vi "SNF_Analog.vi"() -> ()   [LabVIEW 2017]
uses:
  Users/Darcy/Documents/LabVIEW Data/MathScriptVIs/MCStatic_38597428832_1f828b6118eee4aae6c26f87bca7dc42.vi
  <instcachedir>/0/MCStatic_38597428832_1f828b6118eee4aae6c26f87bca7dc42_D4E3D0E3241540FEBE7742005F22DD6C.lvgen/MCStatic_38597428832_1f828b6118eee4aae6c26f87bca7dc42_D4E3D0E3241540FEBE7742005F22DD6C_001.vi
  <vilib>/imath/engines/lvmath2/RunTimeEngine/IndexRead/NIMS V(S).vi
  <instcachedir>/0/NIMS V(S)_0488751826AF41519A22953C041130DC.lvgen/NIMS V(S)_0488751826AF41519A22953C041130DC_000.vi
  <vilib>/imathl/engines/lvmath/Functions/Error Handling/Create Error.vi
  <vilib>/imath/engines/lvmath2/RunTimeEngine/NodeEndStatement/NIMS_NodeEndStatement_Output.vi
  <instcachedir>/0/NIMS_NodeEndStatement_Output_53EC0D466D134D7ABD903AC30B43404B.lvgen/NIMS_NodeEndStatement_Output_53EC0D466D134D7ABD903AC30B43404B_001.vi
  <instcachedir>/0/NIMS_NodeEndStatement_Output_53EC0D466D134D7ABD903AC30B43404B.lvgen/NIMS_NodeEndStatement_Output_53EC0D466D134D7ABD903AC30B43404B_005.vi
  <vilib>/imath/engines/lvmath2/RunTimeEngine/ErrorHandling/NIMS_Finalize Error.vi
  <vilib>/Utility/file.llb/Read Delimited Spreadsheet (DBL).vi
  Users/Darcy/Documents/LabVIEW Data/reactor_power.m
  Users/Darcy/Documents/LabVIEW Data/long_term_power.m
  Users/Darcy/Documents/LabVIEW Data/power_function.m
  Users/Darcy/Documents/LabVIEW Data/short_term_power.m
panel:
  out "Coolant Temp\n Avg.":dbl
  in  "dt (milliseconds)":i64=50
  in  "CRsteady":dbl=50.0 format="%#_13g"
  in  "CRamp":dbl=200.0
  in  "power":dbl=50.0 format="%#_13g"
  in  "P_max: 100":dbl=200.0
  in  "P_min: 1":dbl=1.0
  out "ST Avg.":dbl
  out "Coolant Temp":dbl(slide) scale=20.0..100.0
  out "Fuel Temp":dbl(slide) scale=100.0..175.0
  out "BT Avg.":dbl
  out "CX Avg.":dbl
  in  "Input Length":dbl
  out "Iterations":dbl
  in  "?":bool
  in  "?":bool
  out "Array":dbl[](array[numeric])
  in  "INPUT/MANUAL":bool
  in  "Load Power Profile":bool
  in  "Dyn. Control Rod Profile File":path
  in  "?":bool
  in  "Equilibrium T_Coolant\nFHR: 100":dbl=100.0
  in  "Equilibrium T_Fuel\nFHR: 100":dbl=100.0
  in  "Coolant Feedback Coef\nFHR: -2.1":dbl=-2.1
  in  "Fuel Feedback Coef\nFHR: -6.7":dbl=-6.7
  in  "CRW Coef":dbl=0.005
  in  "CRW Constant":dbl=0.997
  in  "beta\nFHR: 0.0065":dbl=0.0065
  in  "Lambda\nFHR: 5.02e-4":dbl=0.000502
  in  "lambda\nFHR: 0.0785":dbl=0.0785
  out "Net Reactivity":dbl
  out "Rod Reactivity":dbl
  out "Rod 1 In":dbl(slide)
  out "Rod 1 Out":dbl(slide) scale=0.0..1.0
  out "?":dbl(slide) scale=1.0..10000.0
  out "Net Amount Rod Out":dbl
  out "Power [W]":dbl
  in  "SCRAM":bool
  out "Power":dbl(graph)
  out "Resolution 1":dbl=0.05
  out "Control Rod 1 Out":dbl=0.6
  in  "STOP TOGGLE":bool
  # "Neutronics"
  # "Control Rod Worth (CRW)"
  # "Outside Core"
  # "Inside Core"
  # "Temperature Feedback"
  # "Fine"
  # "Input"
  # "Manual"
  # "Coarse"
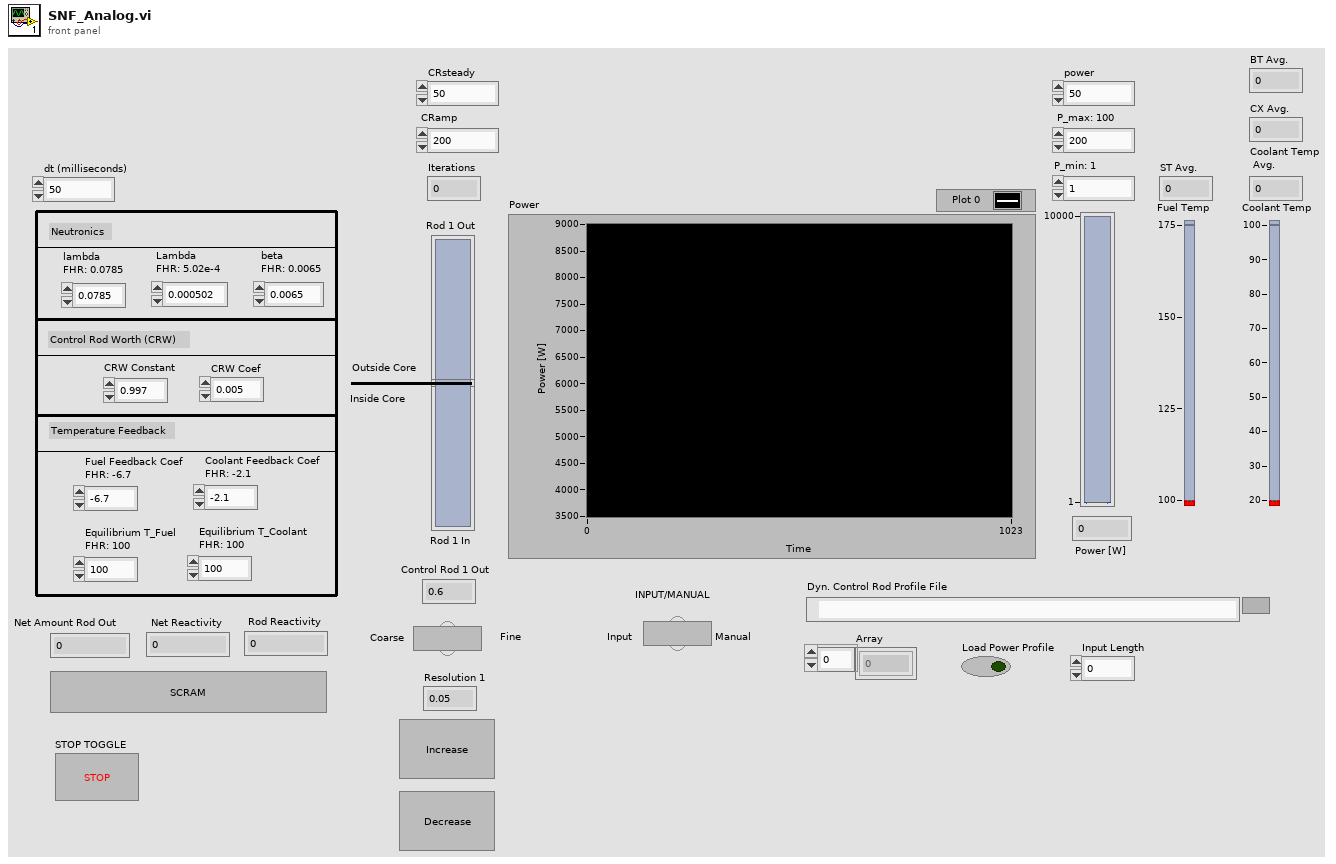
[diagram p1: front panel]
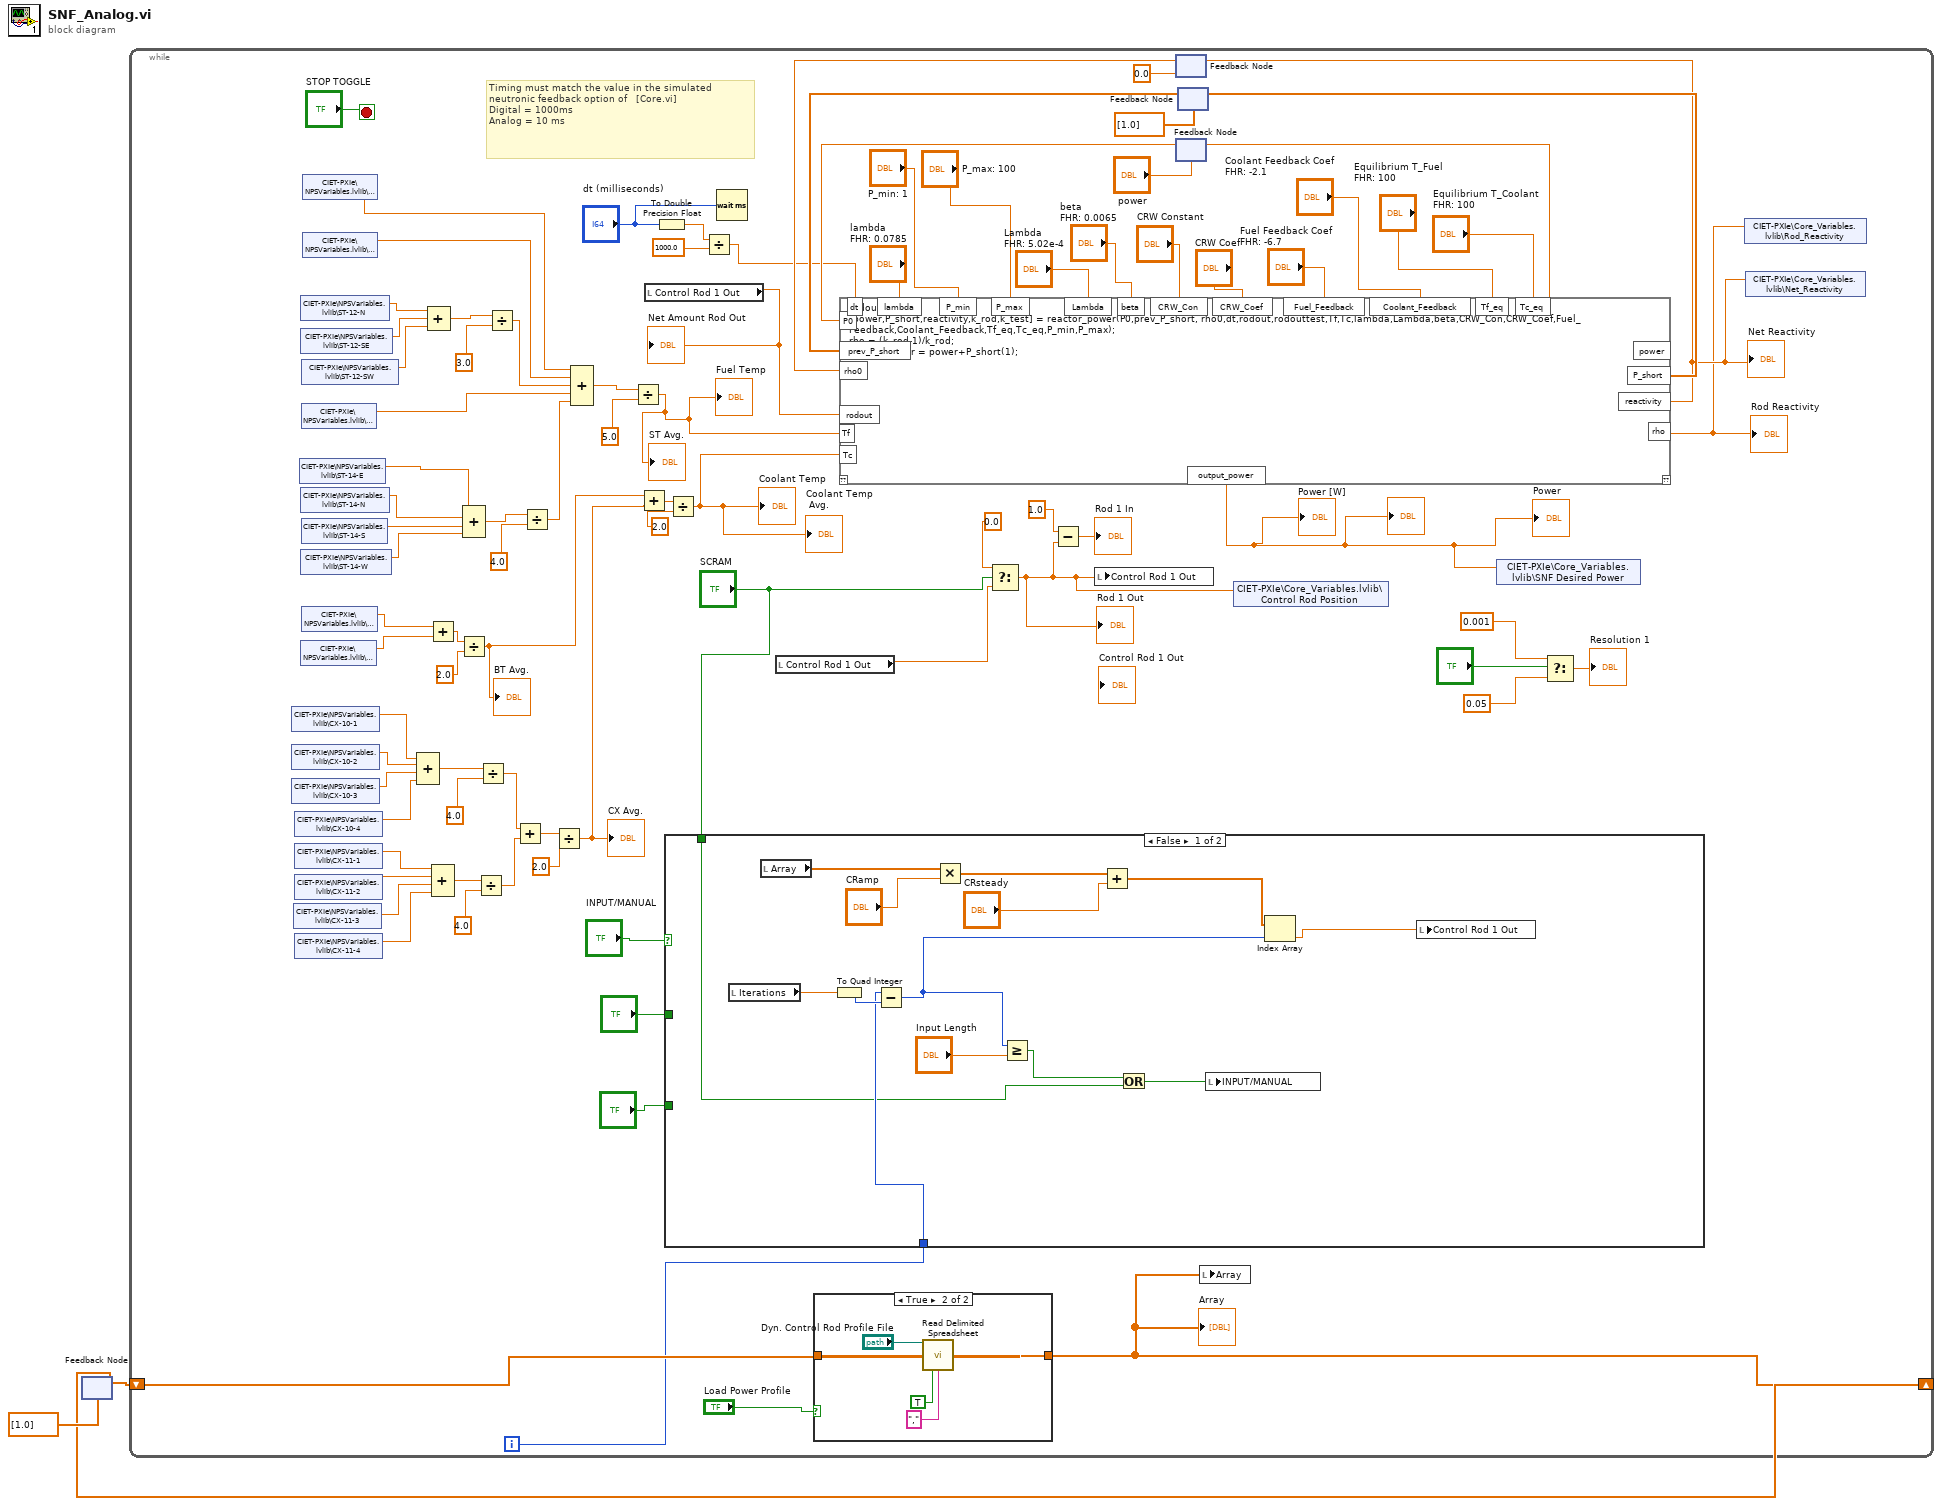
[diagram p0: block diagram]
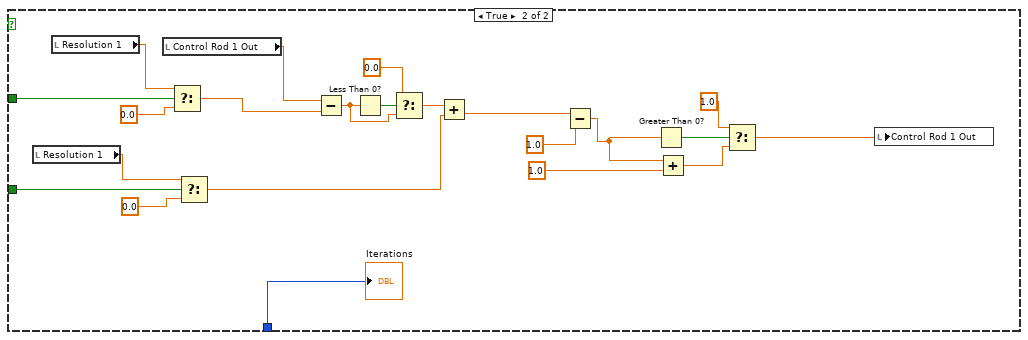
[diagram p2: hidden frame]
diagram:
  n1 = feedback #1(dbl[] [1.0] ("P_short")) -> (w3:dbl[])
  n2 = while {
    shift-right: [w64] -> w1
    shift-left: w3 -> [w65]
    i -> [w59]
    stop <- "STOP TOGGLE" stop-if-true
    # "Timing must match the value in the simulated neutronic feedback option of   [Core.vi] \nDigital = 1000ms \nAnalog = 10 ms"
    n3 = shared-variable "CIET-PXIe\\NPSVariables.lvlib\\CX-10-1"() -> (w24:sgl)  [unwired: 1 in, 1 out]
    n4 = shared-variable "CIET-PXIe\\NPSVariables.lvlib\\CX-10-2"() -> (w23:sgl)  [unwired: 1 in, 1 out]
    n5 = shared-variable "CIET-PXIe\\NPSVariables.lvlib\\CX-10-3"() -> (w22:sgl)  [unwired: 1 in, 1 out]
    n6 = shared-variable "CIET-PXIe\\NPSVariables.lvlib\\CX-11-3"() -> (w18:sgl)  [unwired: 1 in, 1 out]
    n7 = shared-variable "CIET-PXIe\\NPSVariables.lvlib\\CX-10-4"() -> (w21:sgl)  [unwired: 1 in, 1 out]
    n8 = shared-variable "CIET-PXIe\\NPSVariables.lvlib\\CX-11-1"() -> (w20:sgl)  [unwired: 1 in, 1 out]
    n9 = shared-variable "CIET-PXIe\\NPSVariables.lvlib\\CX-11-2"() -> (w19:sgl)  [unwired: 1 in, 1 out]
    n10 = shared-variable "CIET-PXIe\\NPSVariables.lvlib\\CX-11-4"() -> (w17:sgl)  [unwired: 1 in, 1 out]
    n11 = shared-variable "CIET-PXIe\\NPSVariables.lvlib\\ST-14-E"() -> (w39:sgl)  [unwired: 1 in, 1 out]
    n12 = shared-variable "CIET-PXIe\\NPSVariables.lvlib\\ST-12-N"() -> (w46:sgl)  [unwired: 1 in, 1 out]
    n13 = shared-variable "CIET-PXIe\\NPSVariables.lvlib\\ST-12-SE"() -> (w45:sgl)  [unwired: 1 in, 1 out]
    n14 = shared-variable "CIET-PXIe\\NPSVariables.lvlib\\ST-14-N"() -> (w38:sgl)  [unwired: 1 in, 1 out]
    n15 = shared-variable "CIET-PXIe\\NPSVariables.lvlib\\ST-14-W"() -> (w36:sgl)  [unwired: 1 in, 1 out]
    n16 = shared-variable "CIET-PXIe\\NPSVariables.lvlib\\BT-12"() -> (w53:sgl)  [unwired: 1 in, 1 out]
    n17 = shared-variable "CIET-PXIe\\NPSVariables.lvlib\\ST-12-SW"() -> (w44:sgl)  [unwired: 1 in, 1 out]
    n18 = shared-variable "CIET-PXIe\\NPSVariables.lvlib\\ST-13"() -> (w42:sgl)  [unwired: 1 in, 1 out]
    n19 = shared-variable "CIET-PXIe\\NPSVariables.lvlib\\ST-14-S"() -> (w37:sgl)  [unwired: 1 in, 1 out]
    n20 = shared-variable "CIET-PXIe\\NPSVariables.lvlib\\BT-11"() -> (w54:sgl)  [unwired: 1 in, 1 out]
    n21 = shared-variable "CIET-PXIe\\NPSVariables.lvlib\\ST-10"() -> (w52:sgl)  [unwired: 1 in, 1 out]
    n22 = shared-variable "CIET-PXIe\\NPSVariables.lvlib\\ST-11"() -> (w51:sgl)  [unwired: 1 in, 1 out]
    n23 = Compound Arithmetic op=ADD(w24, w23, w22, w21) -> (w30:sgl)
    n24 = Compound Arithmetic op=ADD(w46, w45, w44) -> (w48:sgl)
    n25 = Add(x=w54, y=w53) -> (x+y=w56:sgl)
    n26 = Compound Arithmetic op=ADD(w20, w19, w18, w17) -> (w28:sgl)
    n27 = Divide(x=w56, y=2.0) -> (x/y=w33:dbl)
    "BT Avg." <- w33
    n28 = Compound Arithmetic op=ADD(w39, w38, w37, w36) -> (w41:sgl)
    n29 = Divide(x=w28, y=4.0) -> (x/y=w25:dbl)
    n30 = Divide(x=w30, y=4.0) -> (x/y=w26:dbl)
    n31 = Divide(x=w48, y=3.0) -> (x/y=w43:dbl)
    n32 = Add(x=w26, y=w25) -> (x+y=w58:dbl)
    n33 = Divide(x=w41, y=4.0) -> (x/y=w35:dbl)
    n34 = Divide(x=w58, y=2.0) -> (x/y=w32:dbl)
    "CX Avg." <- w32
    n35 = Compound Arithmetic op=ADD(w52, w51, w43, w42, w35) -> (w50:dbl)
    n36 = Divide(x=w50, y=5.0) -> (x/y=w16:dbl)
    "Fuel Temp" <- w16
    "ST Avg." <- w16
    n37 = Add(x=w33, y=w32) -> (x+y=w31:dbl)
    n38 = local read "Control Rod 1 Out"() -> (w67:dbl)
    "Net Amount Rod Out" <- w67
    n39 = To Double Precision Float(number="dt (milliseconds)") -> (double precision float=w7:dbl)
    n40 = case shown="False" "INPUT/MANUAL" {
      tunnel: "?" -> [_ w110]
      tunnel: "?" -> [_ w109]
      tunnel: w59 -> [w102 w108]
      tunnel: "SCRAM" -> [w100 _]
      frame False {
        n41 = local read "Iterations"() -> (w104:dbl)
        n42 = local read "Array"() -> (w97:dbl[])
        n43 = To Quad Integer(1:w104) -> (0:w103:i64)
        n44 = Subtract(x=w102, y=w103) -> (x-y=w105:i64)
        n45 = Multiply(x=w97, y="CRamp") -> (x*y=w95:dbl[])
        n46 = Greater Or Equal?(x=w105, y="Input Length") -> (x >= y?=w101:bool)
        n47 = Add(x=w95, y="CRsteady") -> (x+y=w93:dbl[])
        n48 = Or(x=w101, y=w100) -> (x .or. y?=w99:bool)
        n49 = local write "INPUT/MANUAL"(w99) -> ()
        n50 = Index Array(array=w93, index=w105) -> (element=w98:dbl)
        n51 = local write "Control Rod 1 Out"(w98) -> ()
      }
      frame True {
        n52 = local read "Resolution 1"() -> (w126:dbl)
        n53 = local read "Resolution 1"() -> (w128:dbl)
        n54 = local read "Control Rod 1 Out"() -> (w124:dbl)
        n55 = Select(t=w128, s=w110, f=0.0) -> (s? t:f=w123:dbl)
        n56 = Select(t=w126, s=w109, f=0.0) -> (s? t:f=w111:dbl)
        n57 = Subtract(x=w124, y=w123) -> (x-y=w121:dbl)
        n58 = Less Than 0?(x=w121) -> (x < 0?=w122:bool)
        n59 = Select(t=0.0, s=w122, f=w121) -> (s? t:f=w119:dbl)
        n60 = Add(x=w119, y=w111) -> (x+y=w118:dbl)
        n61 = Subtract(x=w118, y=1.0) -> (x-y=w114:dbl)
        n62 = Greater Than 0?(x=w114) -> (x > 0?=w116:bool)
        n63 = Add(x=w114, y=1.0) -> (x+y=w113:dbl)
        n64 = Select(t=1.0, s=w116, f=w113) -> (s? t:f=w107:dbl)
        n65 = local write "Control Rod 1 Out"(w107) -> ()
        "Iterations" <- w108
      }
    }
    n66 = Divide(x=w31, y=2.0) -> (x/y=w4:dbl)
    "Coolant Temp" <- w4
    "Coolant Temp\n Avg." <- w4
    n67 = Divide(x=w7, y=1000.0) -> (x/y=w8:dbl)
    n68 = Wait (ms)(milliseconds to wait="dt (milliseconds)") -> ()  [unwired: 1 out]
    n69 = local read "Control Rod 1 Out"() -> (w60:dbl)
    n70 = case shown="True" "Load Power Profile" {
      tunnel: [w129 w130] -> w64
      tunnel: w65 -> [w129 _]
      frame False {
      }
      frame True {
        n71 = call-poly <vilib>:"Read Delimited Spreadsheet.vi"("file path (dialog if empty)"="Dyn. Control Rod Profile File", "transpose? (F)"=TRUE, "delimiter (\\t)"="," ("delimiter (\\t)")) -> ("first row"=w130:dbl[])  [unwired: 7 in, 5 out]
      }
    }
    "Array" <- w64
    n72 = Select(t=0.0, s="SCRAM", f=w60) -> (s? t:f=w11:dbl)
    "Rod 1 Out" <- w11
    n73 = Subtract(x=1.0, y=w11) -> (x-y=→"Rod 1 In":dbl)
    n74 = local write "Control Rod 1 Out"(w11) -> ()
    n75 = feedback #2(0.0 ("reactivity")) -> (w84:dbl)
    n76 = feedback #3("power") -> (w87:dbl)
    n77 = feedback #4(dbl[] [1.0] ("P_short")) -> (w85:dbl[])
    n78 = mathscript code="rodouttest = 0;\n[power,P_short,reactivity,k_rod,k_test] = reactor_power(P0,prev_P_short, rho0,dt,rodout,rodouttest,Tf,Tc,lambda,Lambda,beta,CRW_Con,CRW_Coef,Fuel_Feedback,Coolant_Feedback,Tf_eq,Tc_eq,P_min,P_max);\nrho = (k_rod-1)/k_rod;\noutput_power = power+P_short(1);"("rodout"=w67, "P0"=w87, "prev_P_short"=w85, "rho0"=w84, "Tf"=w16, "Tc"=w4, "lambda"="lambda\nFHR: 0.0785", "Lambda"="Lambda\nFHR: 5.02e-4", "beta"="beta\nFHR: 0.0065", "CRW_Con"="CRW Constant", "CRW_Coef"="CRW Coef", "Fuel_Feedback"="Fuel Feedback Coef\nFHR: -6.7", "Coolant_Feedback"="Coolant Feedback Coef\nFHR: -2.1", "Tf_eq"="Equilibrium T_Fuel\nFHR: 100", "Tc_eq"="Equilibrium T_Coolant\nFHR: 100", "P_max"="P_max: 100", "P_min"="P_min: 1", "dt"=w8) -> ("power"=w88:dbl, "P_short"=w86:dbl[], "reactivity"=w10:dbl, "output_power"=w12:dbl, "rho"=w9:dbl)  [unwired: 1 in, 1 out]
    "Power" <- w12
    "Power [W]" <- w12
    "?" <- w12
    "Rod Reactivity" <- w9
    "Net Reactivity" <- w10
    n79 = feedback-in #2(w10) -> ()
    n80 = feedback-in #3(w88) -> ()
    n81 = feedback-in #4(w86) -> ()
    n82 = local write "Array"(w64) -> ()
    n83 = shared-variable "CIET-PXIe\\Core_Variables.lvlib\\Control Rod Position"(w11) -> ()  [unwired: 1 in, 1 out]
    n84 = shared-variable "CIET-PXIe\\Core_Variables.lvlib\\SNF Desired Power"(w12) -> ()  [unwired: 1 in, 1 out]
    n85 = Select(t=0.001, s="?", f=0.05) -> (s? t:f=→"Resolution 1":dbl)
    n86 = shared-variable "CIET-PXIe\\Core_Variables.lvlib\\Rod_Reactivity"(w9) -> ()  [unwired: 1 in, 1 out]
    n87 = shared-variable "CIET-PXIe\\Core_Variables.lvlib\\Net_Reactivity"(w10) -> ()  [unwired: 1 in, 1 out]
  }
  n88 = feedback-in #1(w1) -> ()
